vi "PulseRateCalc.vi"(10 "ResetRate":bool, 11 "TriggerIn":bool) -> (3 "RateOut":fxp<+/-,64,32>)   [LabVIEW 2014]
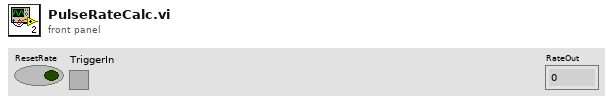
[diagram p1: front panel]
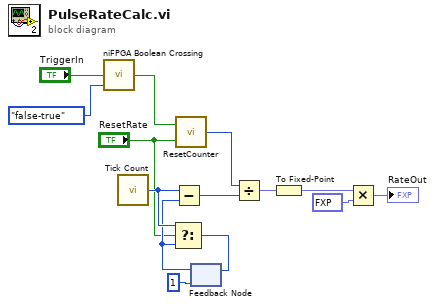
[diagram p0: block diagram]
diagram:
  n1 = call <vilib>:"niFPGA Boolean Crossing.vi"("input"="TriggerIn", "direction"=enum8{"either", "false-true", "true-false"}."false-true") -> ("crossing"=w14:bool)  [unwired: 7 in]
  n2 = call "Tick Count"() -> ("Tick Count(mSec)"=w13:u32)
  n3 = call "ResetCounter.vi"("Reset"="ResetRate", "Increment"=w14) -> ("x+1"=w9:u16)
  n4 = feedback #1(u32 1 ("Tick Count(mSec)")) -> (w11:u32)
  n5 = Select(t=w13, s="ResetRate", f=w11) -> (s? t:f=w12:u32)
  n6 = Subtract(x=w13, y=w11) -> (x-y=w8:u32)
  n7 = feedback-in #1(w12) -> ()
  n8 = Divide(x=w9, y=w8) -> (x/y=w5:fxp<+/-,32,16>)
  n9 = To Fixed-Point(number=w5) -> (fixed-point=w7:fxp<+/-,32,16>)  [unwired: 1 in]
  n10 = Multiply(x=w7, y=fxp<+/-,32,16> 1000.0) -> (x*y=→"RateOut":fxp<+/-,64,32>)
